vi "sine_generation.vi"() -> ()   [LabVIEW 2026]
uses:
  <instrlib>/niUSRP/niUSRP Write Tx Data (CDB).vi
panel:
  in  "IP ADDRESS":refnum<k15>
  in  "waveform size":dbl
  in  "stop":bool
  out "error out":errorcluster
  out "coerced gain":dbl format="%#_6f"
  out "coerced carrier frequency":dbl=100000.0 format="%#_6p"
  out "coerced IQ rate":dbl=100000.0 format="%#_6p"
  in  "active antenna":string
  in  "gain":dbl format="%#_6f"
  in  "carrier frequency":dbl=100000.0 format="%#_6p"
  in  "IQ rate":dbl=100000.0 format="%#_6p"
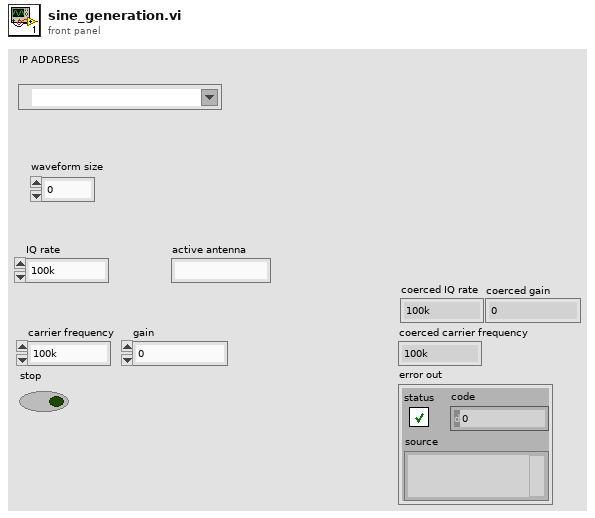
[diagram p1: front panel]
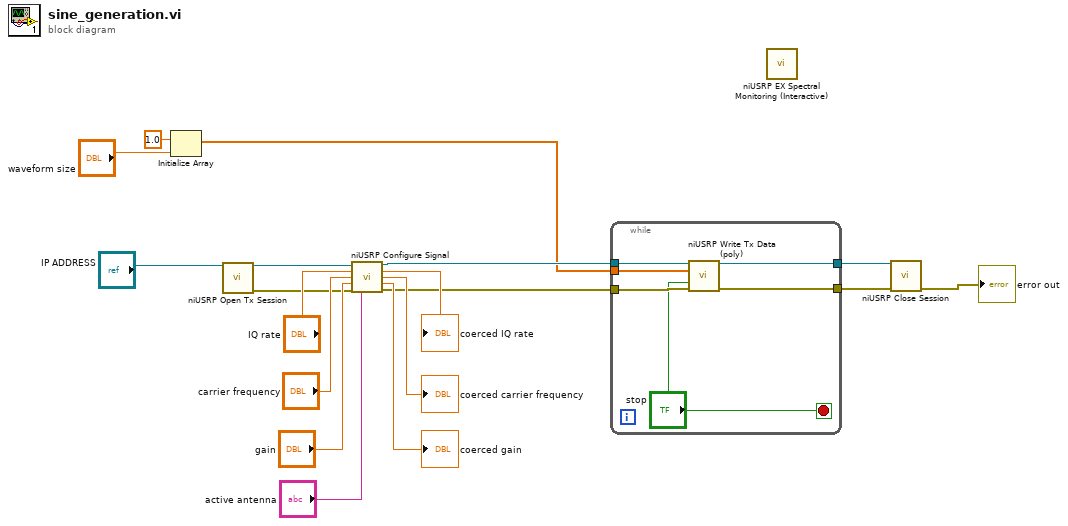
[diagram p0: block diagram]
diagram:
  n1 = Initialize Array(1.0 ("element"), "waveform size") -> (w2:dbl[])
  n2 = call <instrlib>:"niUSRP Open Tx Session.vi"("device names"="IP ADDRESS") -> ("session handle out"=w18:refnum<k15>, "error out"=w10:errorcluster)  [unwired: 13 in]
  n3 = call <instrlib>:"niUSRP Configure Signal.vi"("session handle"=w18, "IQ rate"="IQ rate", "carrier frequency"="carrier frequency", "gain"="gain", "error in (no error)"=w10, "active antenna"="active antenna") -> ("session handle out"=w6:refnum<k15>, "coerced IQ rate"=→"coerced IQ rate":dbl, "coerced carrier frequency"=→"coerced carrier frequency":dbl, "coerced gain"=→"coerced gain":dbl, "error out"=w9:errorcluster)  [unwired: 5 in]
  n4 = while {
    tunnel: w9 -> [w24]
    tunnel: [w23] -> w8
    tunnel: w6 -> [w22]
    tunnel: [w20] -> w5
    tunnel: w2 -> [w19]
    stop <- "stop" stop-if-true
    n5 = call-poly <instrlib>:"niUSRP Write Tx Data (poly).vi"("session handle"=w22, "data"=w19, "end of data?"="stop", "error in (no error)"=w24) -> ("session handle out"=w20:refnum<k15>, "error out"=w23:errorcluster)  [unwired: 10 in]
  }
  n6 = call "niUSRP EX Spectral Monitoring (Interactive).vi"() -> ()  [unwired: 1 in]
  n7 = call <instrlib>:"niUSRP Close Session.vi"("session handle"=w5, "error in (no error)"=w8) -> ("error out"=→"error out":errorcluster)  [unwired: 13 in]
